vi "AKD Get Position Feedback.vi"(0 "connection ID":refnum<k5>, 11 "error in":errorcluster) -> (4 "TCP Refnum":refnum<k5>, 8 "Position (mm)":sgl, 15 "error out":errorcluster)   [LabVIEW 2024]
doc: "This VI reads the PL.FB parameter from the AKD in um (unsigned 16-bit integer), as defined in the drive settings, and converts it to a SGL representing the non-integer position feedback value in mm"
uses:
  MODBUS/NI Modbus.llb/MB Ethernet Master Query Read Holding Registers (poly).vi
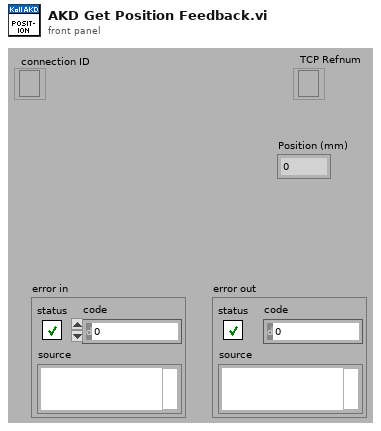
[diagram p1: front panel]
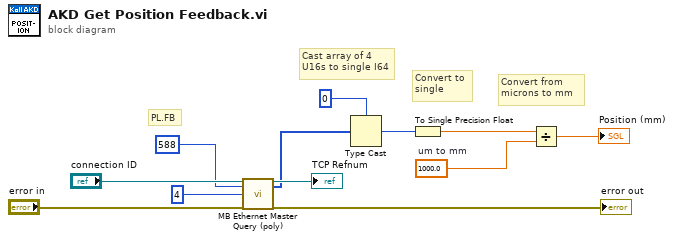
[diagram p0: block diagram]
diagram:
  w2 = sgl 1000.0  # um to mm
  # "Convert from\nmicrons to mm"
  # "Convert to\nsingle"
  # "Cast array of 4\nU16s to single I64"
  # "PL.FB"
  n1 = call-poly "MB Ethernet Master Query (poly).vi"("TCP Connection Refnum in"="connection ID", "Starting Address"=u16 588, "Quantity"=u16 4, "error in"="error in") -> ("TCP Connection Refnum (dup)"=→"TCP Refnum":refnum<k5>, "Holding Registers"=w6:u16[], "error out"=→"error out":errorcluster)  [unwired: 12 in, 1 out]
  n2 = Type Cast(type=i64 0, x=w6) -> (*(type *) &x=w4:i64)
  n3 = To Single Precision Float(number=w4) -> (single precision float=w3:sgl)
  n4 = Divide(x=w3, y=w2) -> (x/y=→"Position (mm)":sgl)
